vi "recursive back.vi"(8 "i":errorcluster, 11 "Value in":refnum<class "Value.lvclass">) -> (0 "error out":errorcluster, 3 "Value out":refnum<class "Value.lvclass">)   [LabVIEW 2023, in "LabGRAD.lvlib" / "Value.lvclass"]
uses:
  Value.lvclass
  Value.lvclass/Value.ctl
  get set ini.ctl
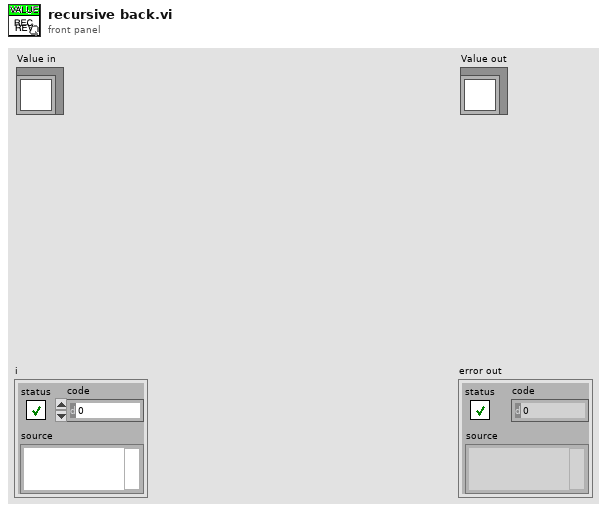
[diagram p1: front panel]
types:
  T1 = typedef "LabGRAD.lvlib/Value.lvclass/get set ini.ctl" = enum16{"get", "set", "ini"}
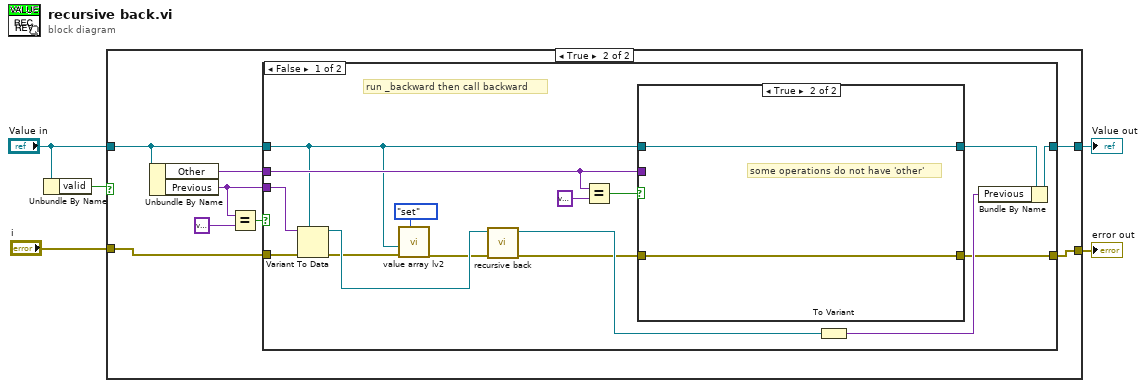
[diagram p0: block diagram]
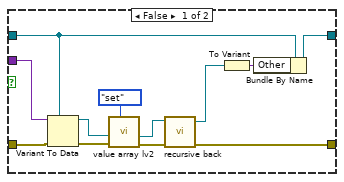
[diagram p3: hidden frame]
diagram:
  n1 = Unbundle By Name("Value in") -> ("valid"=w1:bool)
  n2 = case shown="True" w1 {
    tunnel: [w6 w9] -> w5
    tunnel: [w7 w13] -> w4
    tunnel: "Value in" -> [w7 w14]
    tunnel: "i" -> [w6 w8]
    frame False {
    }
    frame True {
      n3 = Unbundle By Name(w14) -> ("Other"=w15:variant, "Previous"=w10:variant)
      n4 = Equal?(x=w10, y=variant) -> (x = y?=w11:bool)
      n5 = case shown="False" w11 {
        tunnel: w10 -> [w31 _]
        tunnel: w15 -> [w30 _]
        tunnel: w14 -> [w17 w46]
        tunnel: [w26 w46] -> w13
        tunnel: [w22 w47] -> w9
        tunnel: w8 -> [w21 w47]
        frame False {
          # "run _backward then call backward"
          n6 = Variant To Data(error in=w21, type=w17, Variant=w31) -> (data=w20:refnum<class "Value.lvclass">, error out=w19:errorcluster)
          n7 = call "value array lv2.vi"("Enum"=get_set_ini."set", "i"=w19, "Value in"=w17) -> ("out"=w18:errorcluster)  [unwired: 5 in, 2 out]
          n8 = call "recursive back.vi"("i"=w18, "Value in"=w20) -> ("error out"=w23:errorcluster, "Value out"=w25:refnum<class "Value.lvclass">)  [unwired: 8 in]
          n9 = Equal?(x=w30, y=variant) -> (x = y?=w28:bool)
          n10 = case shown="True" w28 {
            tunnel: w17 -> [w42 w45]
            tunnel: w30 -> [w43 _]
            tunnel: [w41 w45] -> w27
            tunnel: w23 -> [w38 w44]
            tunnel: [w37 w44] -> w22
            frame False {
              n11 = Variant To Data(error in=w38, type=w42, Variant=w43) -> (data=w34:refnum<class "Value.lvclass">, error out=w36:errorcluster)
              n12 = call "value array lv2.vi"("Enum"=get_set_ini."set", "i"=w36, "Value in"=w34) -> (0:"out"=w33:errorcluster, 1:"out"=w32:refnum<class "Value.lvclass">)  [unwired: 5 in, 1 out]
              n13 = call "recursive back.vi"("i"=w33, "Value in"=w32) -> ("error out"=w37:errorcluster, "Value out"=w40:refnum<class "Value.lvclass">)  [unwired: 8 in]
              n14 = To Variant(anything=w40) -> (Variant=w39:variant)
              n15 = Bundle By Name(cluster=w42, "Other"=w39) -> (w41:refnum<class "Value.lvclass">)
            }
            frame True {
              # "some operations do not have 'other'"
            }
          }
          n16 = To Variant(anything=w25) -> (Variant=w24:variant)
          n17 = Bundle By Name(cluster=w27, "Previous"=w24) -> (w26:refnum<class "Value.lvclass">)
        }
        frame True {
          # "if no previous, we are finised on this branch"
        }
      }
    }
  }
  "error out" <- w5
  "Value out" <- w4
